vi "PV Software Decode Data.vi"(8 "error in (no error)":errorcluster, 11 "HEX Data (U8)":u8[][](array[numeric]) format="%x") -> (0 "error out":errorcluster, 3 "PV Data":string[][](array[string]))   [LabVIEW 2023]
panel:
  out "Packet Length":u8[](array[numeric])
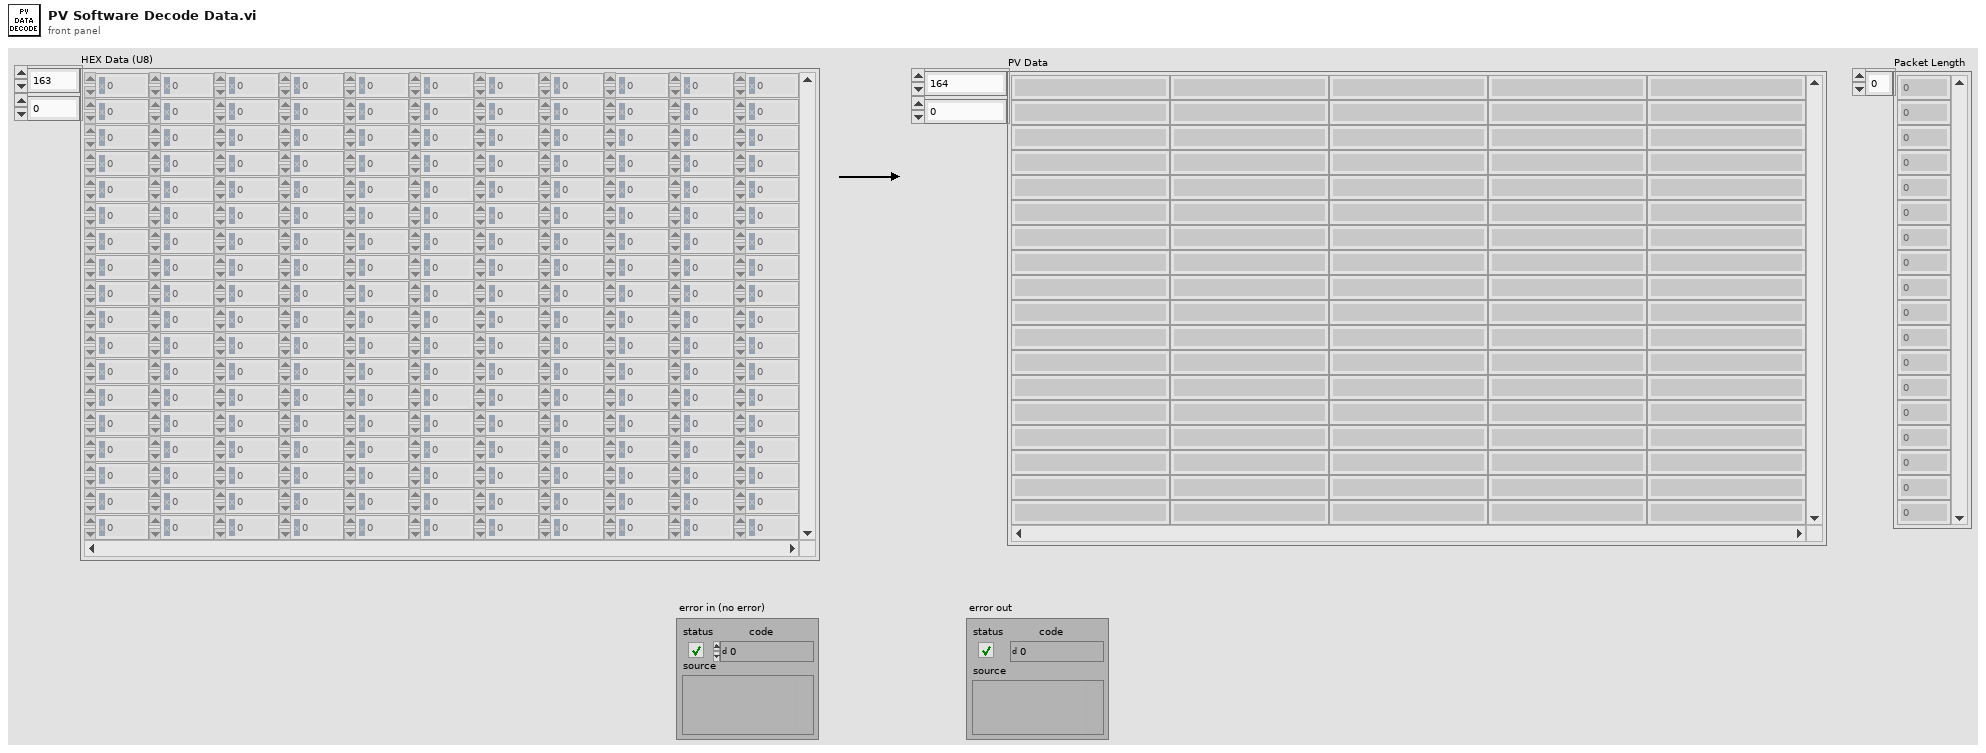
[diagram p1: front panel]
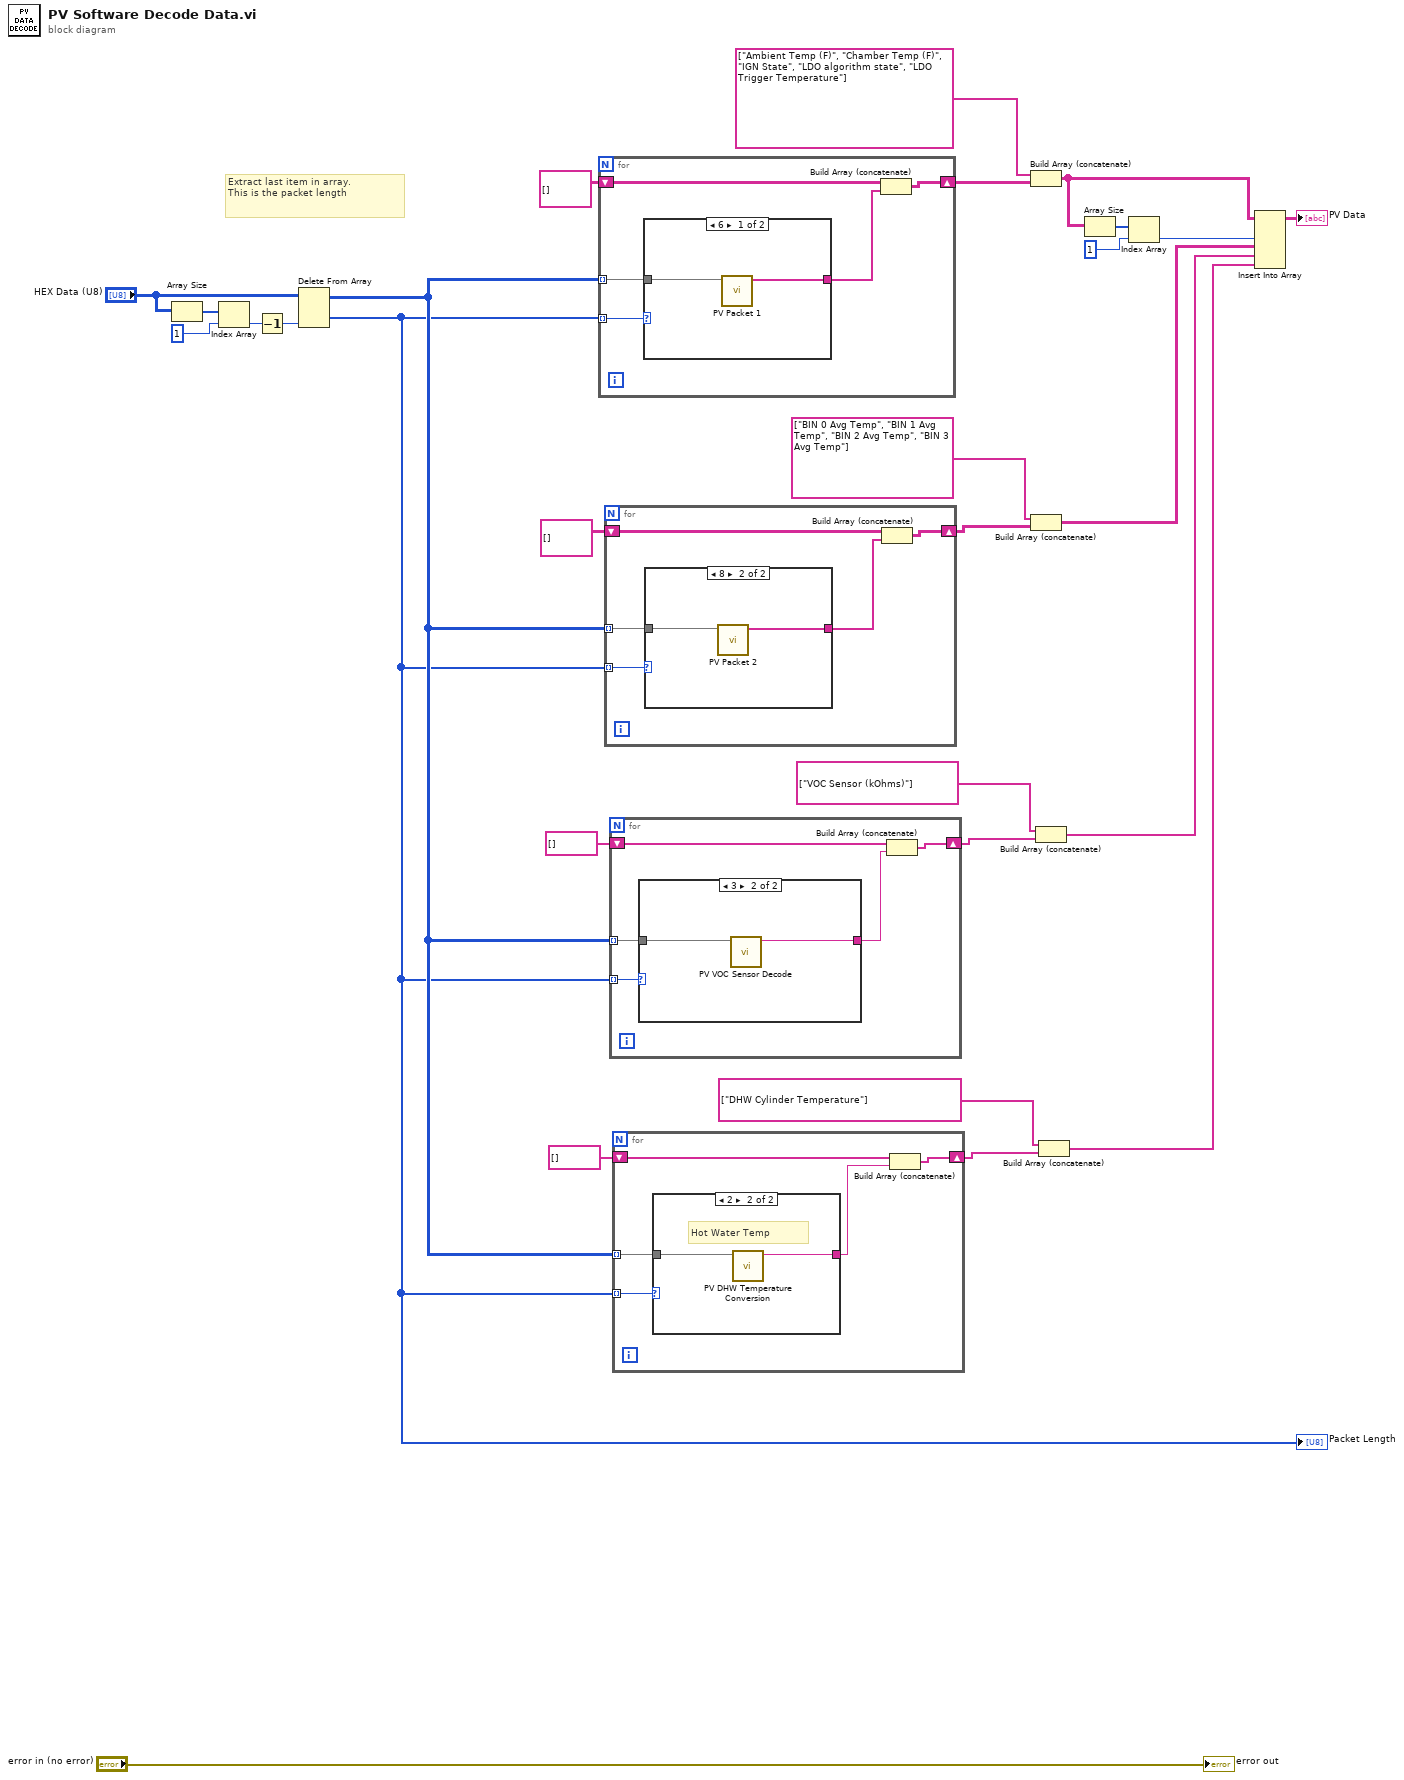
[diagram p0: block diagram]
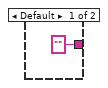
[diagram p2: hidden frame]
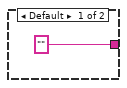
[diagram p3: hidden frame]
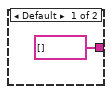
[diagram p4: hidden frame]
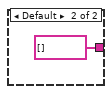
[diagram p5: hidden frame]
diagram:
  # "Extract last item in array. \nThis is the packet length"
  n1 = Array Size(array="HEX Data (U8)") -> (size(s)=w26:i32[])
  n2 = Index Array(array=w26, index=1) -> (element=w24:i32)
  n3 = Decrement(x=w24) -> (x-1=w23:i32)
  n4 = Delete From Array(array="HEX Data (U8)", index (col)=w23) -> (deleted portion=w4:u8[], array with subset deleted=w5:u8[][])  [unwired: 2 in]
  "Packet Length" <- w4
  n5 = for {
    tunnel: w4 -> [w33] mode=indexing
    tunnel: w5 -> [w32] mode=indexing
    shift-right: [w30] -> w19
    shift-left: string[][] [] -> [w31]
    n6 = case shown="6" w33 {
      tunnel: w32 -> [w35 _]
      tunnel: [w34 string[] [] ("PV Data 1")] -> w29
      frame 6 {
        n7 = call "PV Packet 1.vi"("HEX Data (U8) in"=w35) -> ("PV Data 1"=w34:string[])  [unwired: 10 in]
      }
      frame Default {
      }
    }
    n8 = Build Array (concatenate)(w31, w29) -> (w30:string[][])
  }
  n9 = for {
    tunnel: w4 -> [w41] mode=indexing
    tunnel: w5 -> [w40] mode=indexing
    shift-right: [w38] -> w18
    shift-left: string[][] [] -> [w39]
    n10 = case shown="8" w41 {
      tunnel: w40 -> [_ w44]
      tunnel: [string[] [] ("PV Data 2") w43] -> w37
      frame Default {
      }
      frame 8 {
        n11 = call "PV Packet 2.vi"("HEX Data (U8) in"=w44) -> ("PV Data 2"=w43:string[])  [unwired: 10 in]
      }
    }
    n12 = Build Array (concatenate)(w39, w37) -> (w38:string[][])
  }
  n13 = for {
    tunnel: w4 -> [w49] mode=indexing
    tunnel: w5 -> [w48] mode=indexing
    shift-right: [w46] -> w9
    shift-left: string[] [] -> [w47]
    n14 = case shown="3" w49 {
      tunnel: w48 -> [_ w52]
      tunnel: ["" w51] -> w45
      frame Default {
      }
      frame 3 {
        n15 = call "PV VOC Sensor Decode.vi"("HEX Data (U8) in"=w52) -> ("VOC (kOhms)"=w51:string)  [unwired: 10 in]
      }
    }
    n16 = Build Array (concatenate)(w47, w45) -> (w46:string[])
  }
  n17 = for {
    tunnel: w4 -> [w57] mode=indexing
    tunnel: w5 -> [w56] mode=indexing
    shift-right: [w54] -> w1
    shift-left: string[] [] -> [w55]
    n18 = case shown="2" w57 {
      tunnel: w56 -> [_ w60]
      tunnel: ["" ("DHW Temp (°F)") w59] -> w53
      frame Default {
      }
      frame 2 {
        # "Hot Water Temp"
        n19 = call "PV DHW Temperature Conversion.vi"("HEX Data Array (Temp)"=w60) -> ("DHW Temp (°F)"=w59:string)  [unwired: 10 in]
      }
    }
    n20 = Build Array (concatenate)(w55, w53) -> (w54:string[])
  }
  n21 = Build Array (concatenate)(string[] ["Ambient Temp (F)", "Chamber Temp (F)", "IGN State", "LDO algorithm state", "LDO Trigger Temperature"], w19) -> (w15:string[][])
  n22 = Build Array (concatenate)(string[] ["BIN 0 Avg Temp", "BIN 1 Avg Temp", "BIN 2 Avg Temp", "BIN 3 Avg Temp"], w18) -> (w16:string[][])
  n23 = Build Array (concatenate)(string[] ["VOC Sensor (kOhms)"], w9) -> (w3:string[])
  n24 = Build Array (concatenate)(string[] ["DHW Cylinder Temperature"], w1) -> (w2:string[])
  n25 = Array Size(array=w15) -> (size(s)=w14:i32[])
  n26 = Index Array(array=w14, index=1) -> (element=w12:i32)
  n27 = Insert Into Array(array=w15, index (col)=w12, new element #1=w16, new element #2=w3, new element #3=w2) -> (→"PV Data":string[][])  [unwired: 1 in]
  "error out" <- "error in (no error)"
